vi "DB - Get Foreign Keys References.vi"(8 "error in (no error)":errorcluster, 9 "Select":T1(ring), 10 "DB.Schema.Table":string="SRTRS.Config.UnitOfMeasurement", 11 "connection reference":T3) -> (0 "error out":errorcluster, 2 "Foreign Keys References":string[][](array[string]), 3 "connection reference":T3)   [LabVIEW 2013]
uses:
  <vilib>/addons/database/Connection.llb/Conn ObjectReference.ctl
  <vilib>/addons/database/Connection.llb/Conn Execute.vi
  <vilib>/addons/database/Recordset.llb/Rec Fetch Recordset Data (R).vi
  <vilib>/addons/database/Recordset.llb/Rec Destroy - Connection.vi
  <vilib>/addons/database/Connection.llb/DB Tools Open Connec (String).vi
  <vilib>/addons/database/_DB Variant To Data/Database Variant To Data.xnode
  <vilib>/addons/database/NI_Database_API.lvlib
panel:
  out "SQL Query":string
  in  "Connection Information":T2={"Connection "="SQL Server 32bit HPEnvy", "Username"="admin", "Password"="admin123"}
  # "AUTO INTERACTIVE"
  # "Orders\nPartsDetails\nTransactions"
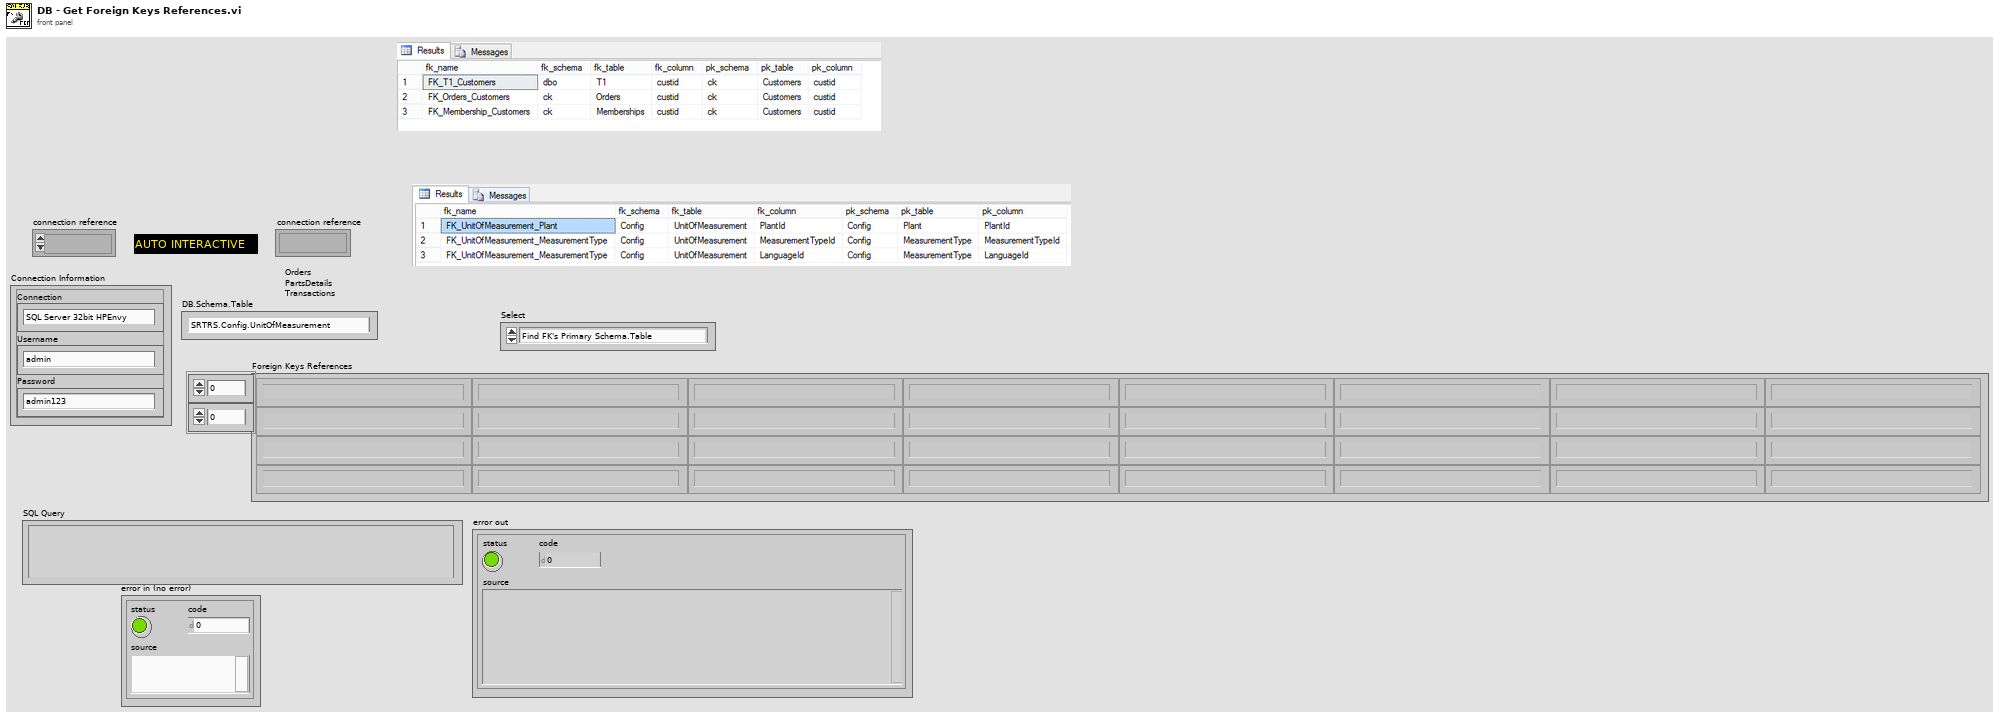
[diagram p1: front panel]
types:
  T1 = enum16{"Find FK's Primary Schema.Table", "Find PK's Foreign Schema.Table"}
  T2 = cluster{"Connection ":string, "Username":string, "Password":string}
  T3 = typedef "NI_Database_API.lvlib/Conn ObjectReference.ctl" = refnum<k1>
  T4 = typedef "Enum - InteractiveMode-SubVIMode.ctl" = enum16{"Interactive", "subVI Mode"}
  T5 = typedef "DB - DB.Schema.Table.ctl" = cluster{"DB":string, "Schema":string, "Table":string}
  T6 = typedef "NI_Database_API.lvlib/Rec ObjectReference.ctl" = refnum<k1>
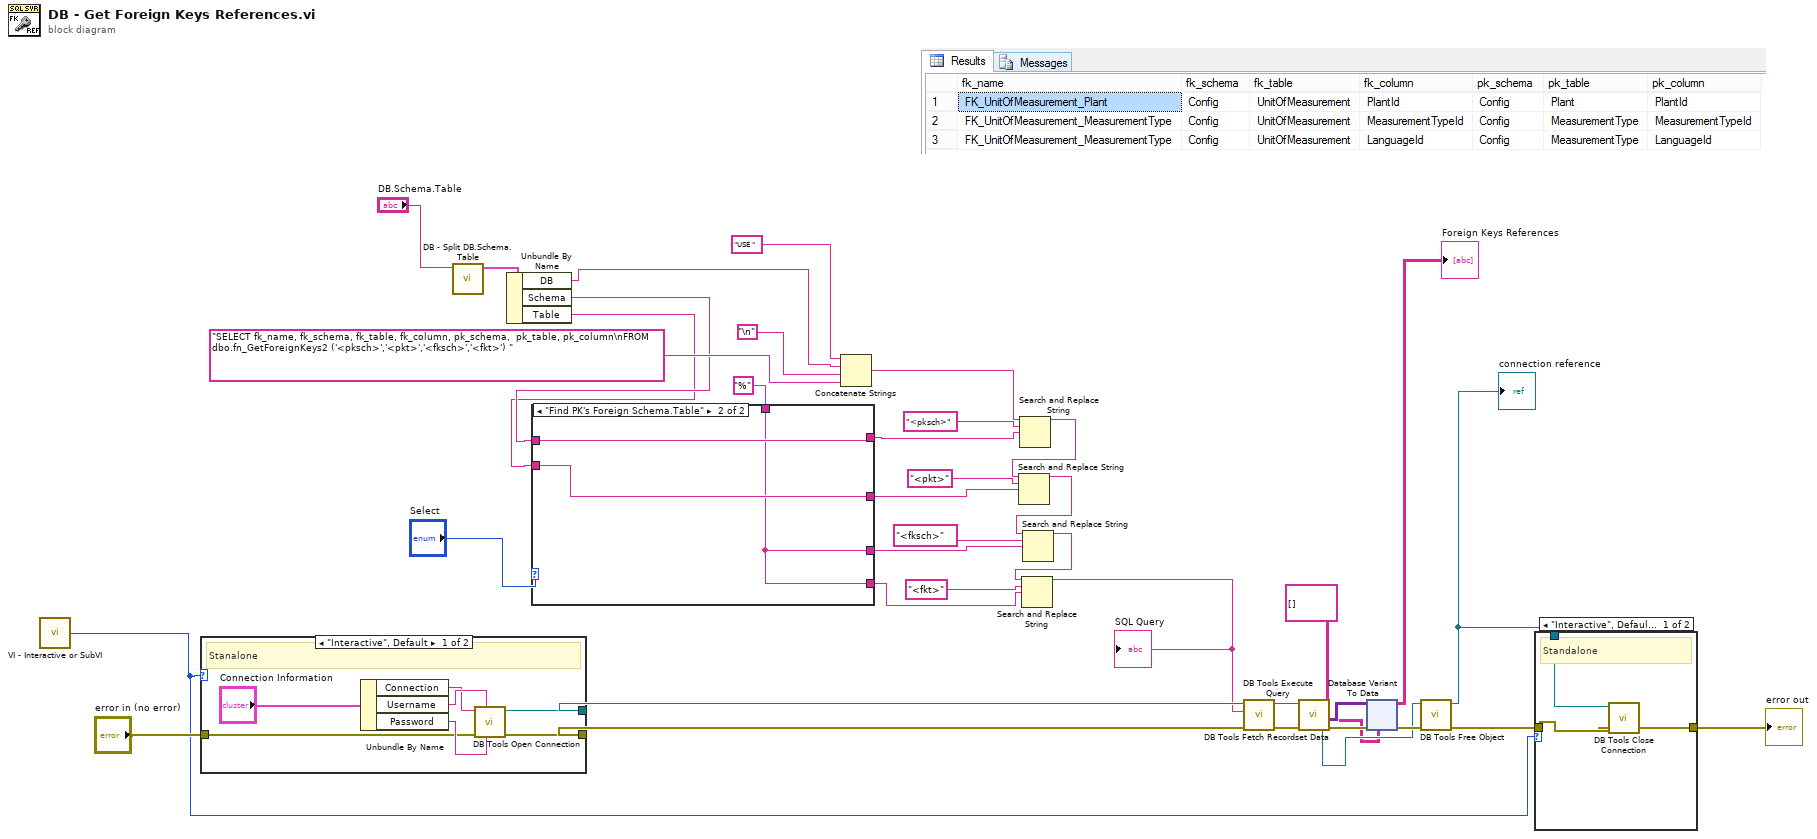
[diagram p0: block diagram]
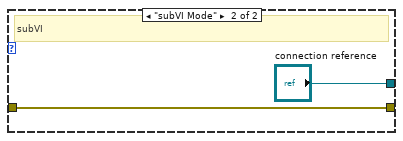
[diagram p4: hidden frame]
diagram:
  n1 = call "VI - Interactive or SubVI.vi"() -> ("Mode"=w1:T4)  [unwired: 5 in]
  n2 = case shown="\"Interactive\", Default" w1 {
    tunnel: [w41 "connection reference"] -> w29
    tunnel: "error in (no error)" -> [w40 w46]
    tunnel: [w39 w46] -> w31
    frame "Interactive", Default {
      # "Stanalone"
      n3 = Unbundle By Name("Connection Information") -> ("Connection"=w43:string, "Username"=w44:string, "Password"=w42:string)
      n4 = call-poly <vilib>:"DB Tools Open Connection.vi"("password"=w42, "userID"=w44, "error in (no error)"=w40, "connection information"=w43) -> ("error out"=w39:errorcluster, "connection reference"=w41:T3)  [unwired: 4 in]
    }
    frame "subVI Mode" {
      # "subVI"
    }
  }
  n5 = call "DB - Split DB.Schema.Table.vi"("DB.Schema.Table"="DB.Schema.Table") -> ("DB.Schema.Table"=w20:T5)  [unwired: 10 in]
  n6 = Unbundle By Name(w20) -> ("DB"=w19:string, "Schema"=w17:string, "Table"=w16:string)
  n7 = case shown="\"Find PK's Foreign Schema.Table\"" "Select" {
    tunnel: w17 -> [w50 w53]
    tunnel: w16 -> [w49 w52]
    tunnel: [w48 w53] -> w7
    tunnel: [w48 w52] -> w6
    tunnel: [w50 w51] -> w5
    tunnel: [w49 w51] -> w4
    tunnel: "%" -> [w48 w51]
    frame "Find FK's Primary Schema.Table", Default {
    }
    frame "Find PK's Foreign Schema.Table" {
    }
  }
  n8 = Concatenate Strings("USE ", w19, "\n", "SELECT fk_name, fk_schema, fk_table, fk_column, pk_schema,  pk_table, pk_column\nFROM dbo.fn_GetForeignKeys2 ('<pksch>','<pkt>','<fksch>','<fkt>') " ("string")) -> (w15:string)
  n9 = Search and Replace String(input string=w15, search string="<pksch>" ("string"), replace string=w7) -> (result string=w14:string)  [unwired: 5 in, 3 out]
  n10 = Search and Replace String(input string=w14, search string="<pkt>" ("string"), replace string=w6) -> (result string=w13:string)  [unwired: 5 in, 3 out]
  n11 = Search and Replace String(input string=w13, search string="<fksch>" ("string"), replace string=w5) -> (result string=w12:string)  [unwired: 5 in, 3 out]
  n12 = Search and Replace String(input string=w12, search string="<fkt>" ("string"), replace string=w4) -> (result string=w2:string)  [unwired: 5 in, 3 out]
  "SQL Query" <- w2
  n13 = call-poly <vilib>:"DB Tools Execute Query.vi"("error in (no error)"=w31, "SQL query"=w2, "connection reference"=w29) -> ("error out"=w35:errorcluster, "recordset reference"=w33:T6)  [unwired: 5 in]
  n14 = call-poly <vilib>:"DB Tools Fetch Recordset Data.vi"("error in (no error)"=w35, "recordset reference"=w33) -> ("error out"=w37:errorcluster, "recordset data"=w36:variant[][], "recordset reference out"=w34:T6)  [unwired: 3 in]
  n15 = xnode "Database Variant To Data"("database variant"=w36, "error in (no error)"=w37, "type"=string[][] []) -> ("data"=→"Foreign Keys References":string[][], "error out"=w38:errorcluster)
  n16 = call-poly <vilib>:"DB Tools Free Object.vi"("error in (no error)"=w38, "recordset reference"=w34) -> ("error out"=w27:errorcluster, "connection reference"=w25:T3)  [unwired: 8 in]
  "connection reference" <- w25
  n17 = case shown="\"Interactive\", Default" w1 {
    tunnel: w25 -> [w56 _]
    tunnel: w27 -> [w55 w57]
    tunnel: [w54 w57] -> w28
    frame "Interactive", Default {
      # "Standalone"
      n18 = call <vilib>:"DB Tools Close Connection.vi"("error in (no error)"=w55, "connection reference"=w56) -> ("error out"=w54:errorcluster)  [unwired: 5 in]
    }
    frame "subVI Mode" {
      # "subVI"
    }
  }
  "error out" <- w28
